vi "ukol3.vi"() -> ()   [LabVIEW 2023]
uses:
  <vilib>/Utility/file.llb/Read Delimited Spreadsheet (DBL).vi
  <vilib>/Analysis/NI_AALPro.lvlib
panel:
  out "Waveform Graph 2":waveform(dbl)[](graph)
  out "subarray":dbl[](array[numeric])
  out "Waveform Graph":waveform(dbl)(graph)
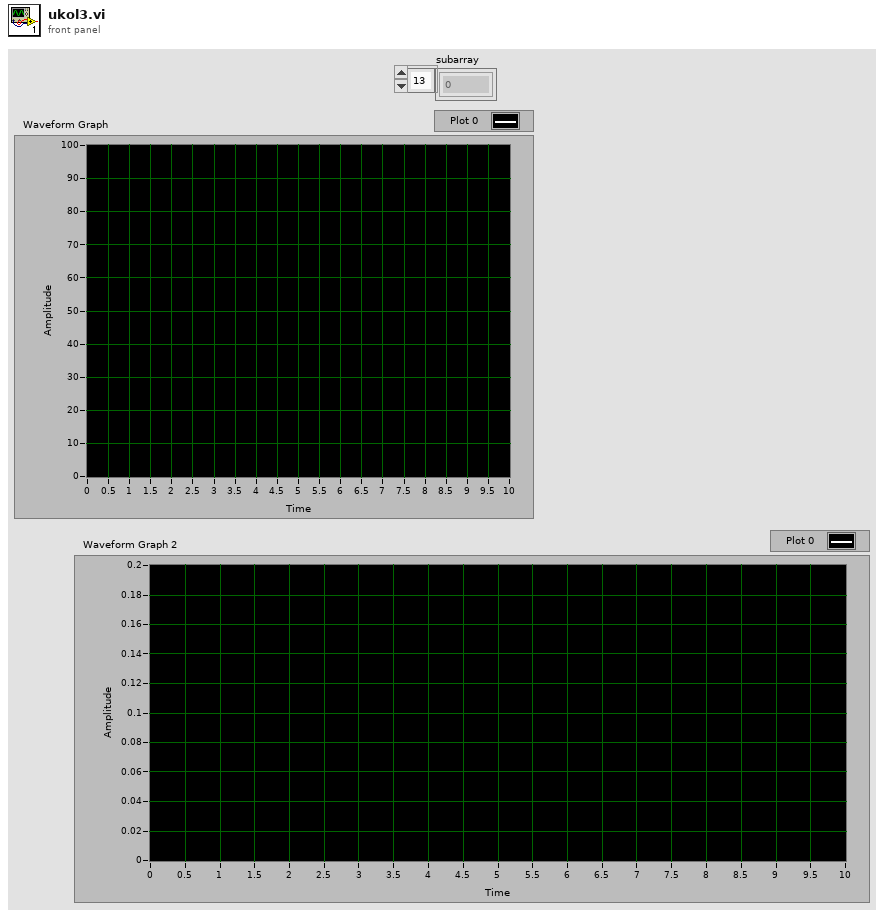
[diagram p1: front panel]
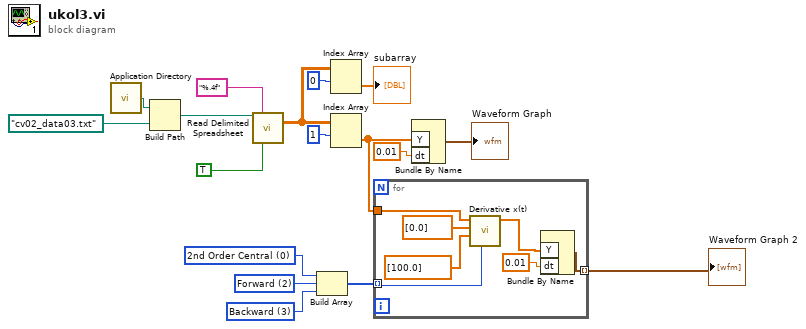
[diagram p0: block diagram]
diagram:
  w3 = u16 3 items=["2nd Order Central", "4th Order Central", "Forward", "Backward"] ("method")
  w4 = u16 2 items=["2nd Order Central", "4th Order Central", "Forward", "Backward"] ("method")
  w5 = u16 0 items=["2nd Order Central", "4th Order Central", "Forward", "Backward"] ("method")
  n1 = call <vilib>:"Application Directory.vi"() -> ("Application Directory"=w17:path)
  n2 = Build Path(base path=w17, name or relative path=path "cv02_data03.txt") -> (appended path=w15:path)
  n3 = call-poly <vilib>:"Read Delimited Spreadsheet.vi"("file path (dialog if empty)"=w15, "format (%.3f)"="%.4f", "transpose? (F)"=TRUE) -> ("all rows"=w10:dbl[][])  [unwired: 7 in, 5 out]
  n4 = Build Array(w5, w4, w3) -> (w2:u16[])
  n5 = Index Array(array=w10, index (row)=0) -> (element=→"subarray":dbl[])  [unwired: 1 in]
  n6 = Index Array(array=w10, index (row)=1) -> (element=w6:dbl[])  [unwired: 1 in]
  n7 = for {
    tunnel: w6 -> [w24]
    tunnel: w2 -> [w23] mode=indexing
    tunnel: [w18] -> w1 mode=indexing
    n8 = call <vilib>:"Derivative x(t).vi"("method"=w23, "Final Condition"=dbl[] [100.0], "Initial Condition"=dbl[] [0.0], "X"=w24) -> ("dX/dt"=w20:dbl[])  [unwired: 6 in, 1 out]
    n9 = Bundle By Name("Y"=w20, "dt"=0.01) -> (w18:waveform(dbl))  [unwired: 1 in]
  }
  "Waveform Graph 2" <- w1
  n10 = Bundle By Name("Y"=w6, "dt"=0.01) -> (→"Waveform Graph":waveform(dbl))  [unwired: 1 in]
